vi "Update Gate Parameters Visibility v2.vi"(7 "Edit User-defined Gate":refnum<vi>, 10 "error in (no error)":errorcluster, 11 "Phasor Explorer Gate Parameters in":refnum<vi>) -> (2 "error out":errorcluster, 3 "Phasor Explorer Gate Parameters out":refnum<vi>)   [LabVIEW 2019]
uses:
  Phasor Explorer Gate Parameters.ctl
  Gate Type.ctl
panel:
  in  "Type of User-defined Function":enum32{"Gate", "IRF"}(radio)
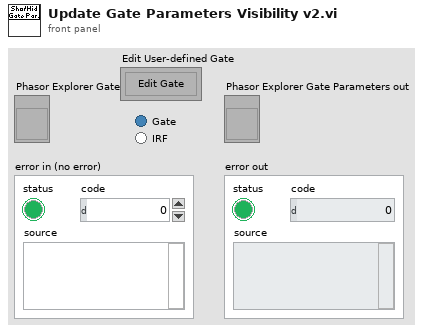
[diagram p1: front panel]
types:
  T1 = typedef "Phasor Explorer Gate Parameters.ctl" = cluster{"First Gate Start":dbl[unit], "Use Gate Center":bool, "Gate Width":dbl[unit], "Gate Step":dbl[unit], "# Gates":dbl, "Gate Type":T2, "Edge Width":dbl[unit], "Top Slope":dbl[unit], "Reversed Sawtooth?":bool, "Analytical Computation":bool, "Integration":enum32{"Item 0", "Item 1"}, "Tolerance":dbl, "# Steps":dbl, "Type of User-defined Function":enum32{"Gate", "IRF"}, "Use Gate Step":bool}
  T2 = typedef "Gate Type.ctl" = enum16{"Square", "Finite Edge Square", "Finite Edge, Tilted Top Square", "Triangle", "Sawtooth", "User-defined"}
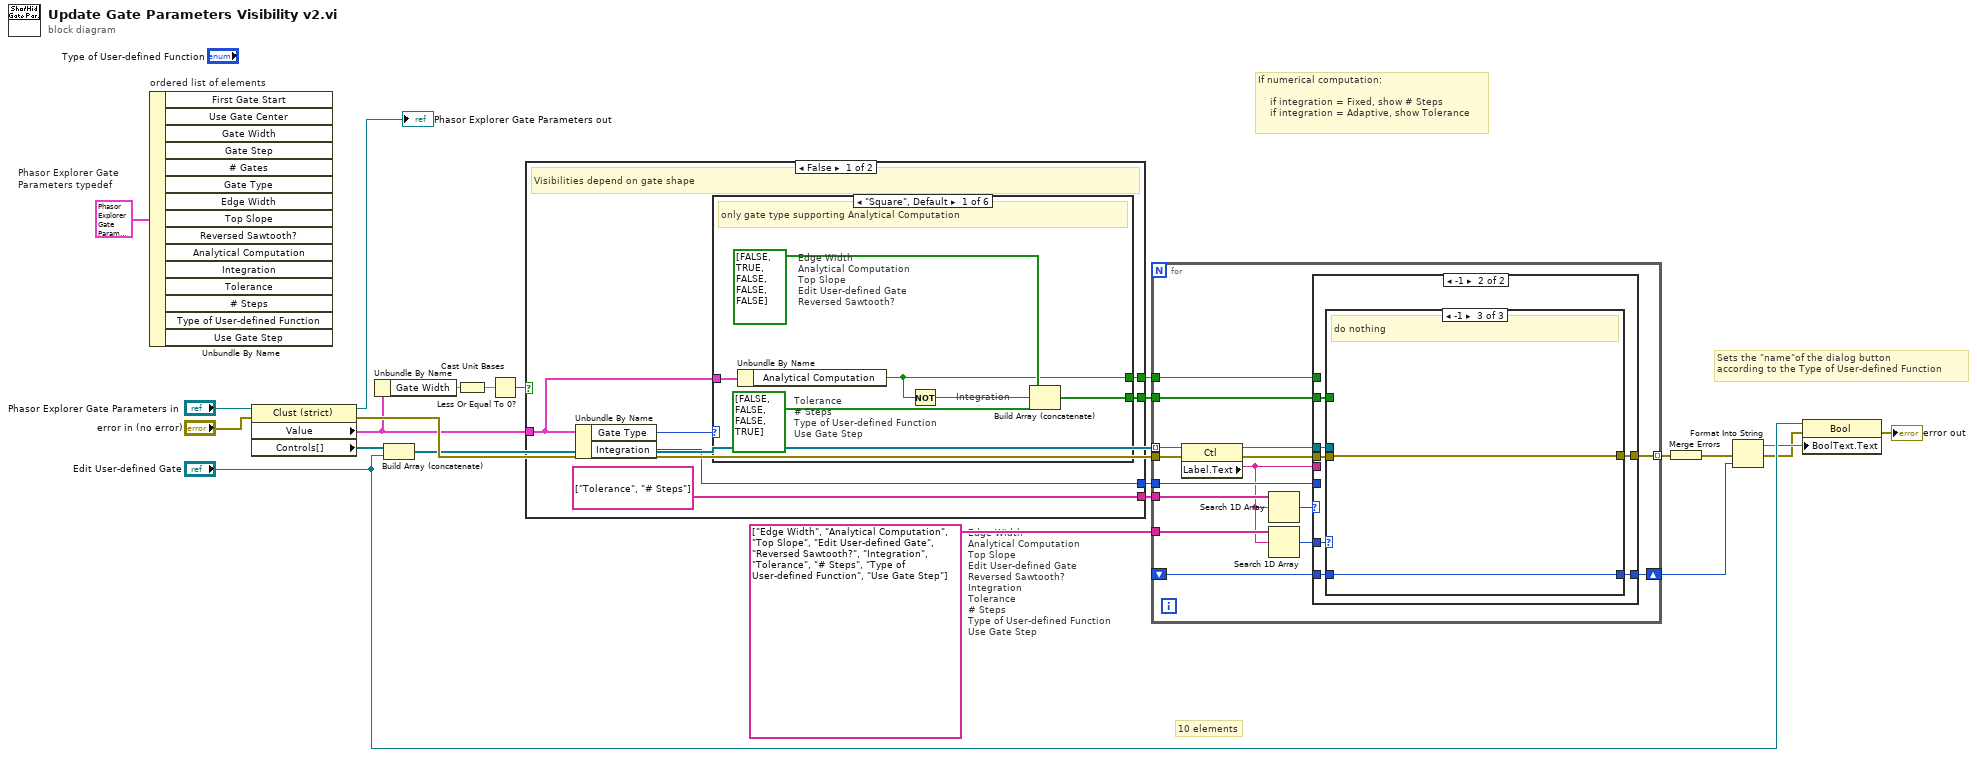
[diagram p0: block diagram]
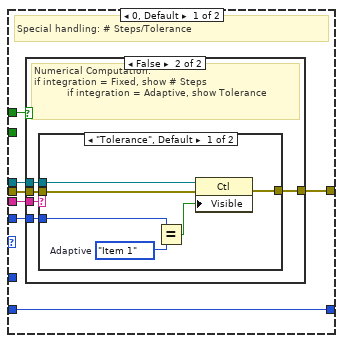
[diagram p2: hidden frame]
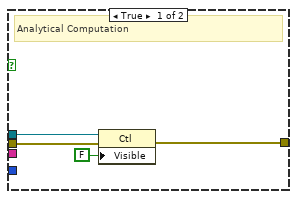
[diagram p3: hidden frame]
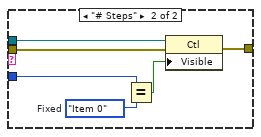
[diagram p4: hidden frame]
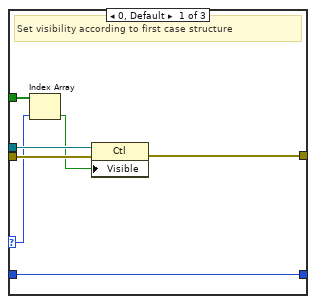
[diagram p5: hidden frame]
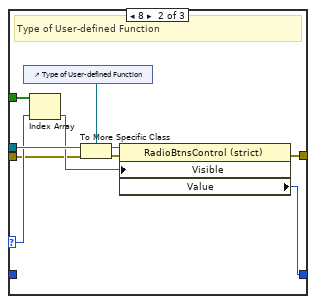
[diagram p6: hidden frame]
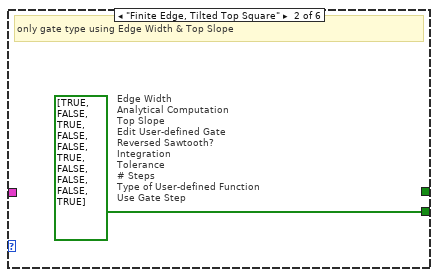
[diagram p7: hidden frame]
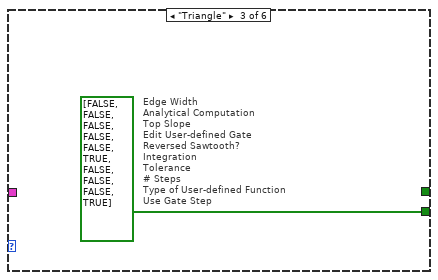
[diagram p8: hidden frame]
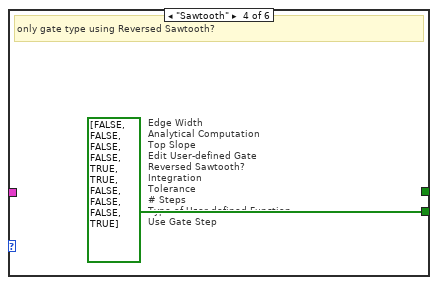
[diagram p9: hidden frame]
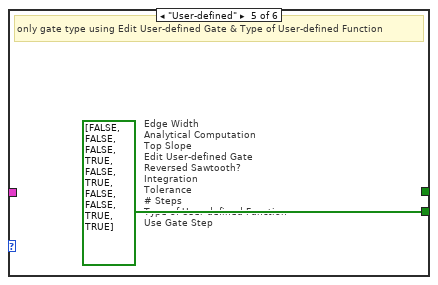
[diagram p10: hidden frame]
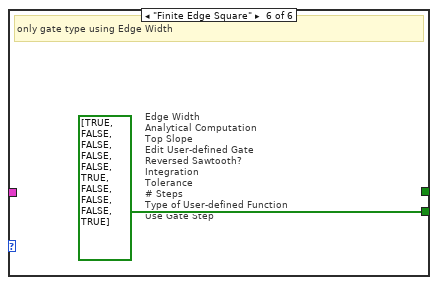
[diagram p11: hidden frame]
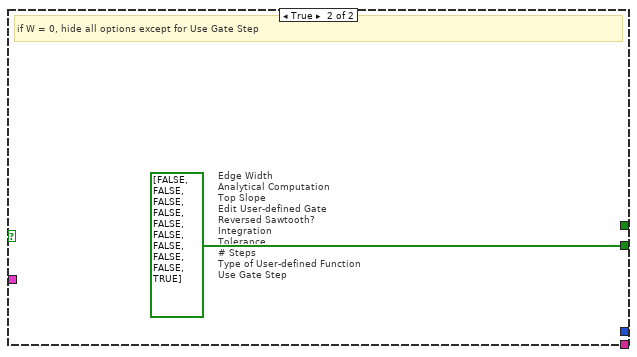
[diagram p12: hidden frame]
diagram:
  w2 = T1 {"First Gate Start"=0.0, "Use Gate Center"=FALSE, "Gate Width"=0.0, "Gate Step"=0.0, "# Gates"=1.0, "Gate Type"=enum."Square", "Edge Width"=0.0, "Top Slope"=0.0, "Reversed Sawtooth?"=FALSE, "Analytical Computation"=FALSE, "Integration"=enum."Item 0", "Tolerance"=1.0, "# Steps"=1.0, "Type of User-defined Function"=enum."Gate", "Use Gate Step"=FALSE}  # Phasor Explorer Gate Parameters typedef
  # "Sets the \"name\"of the dialog button\naccording to the Type of User-defined Function"
  # "If numerical computation:\n\n    if integration = Fixed, show # Steps\n    if integration = Adaptive, show Tolerance"
  # "Edge Width\nAnalytical Computation\nTop Slope\nEdit User-defined Gate\nReversed Sawtooth?\nIntegration\nTolerance\n# Steps\nType of User-defined Function\nUse Gate Step"
  # "10 elements"
  n1 = Unbundle By Name "ordered list of elements"(w2) -> ()  [unwired: 15 out]
  n2 = property class="Clust (strict)"(reference="Phasor Explorer Gate Parameters in", error in="error in (no error)") -> (reference out=→"Phasor Explorer Gate Parameters out":refnum<vi>, error out=w18:errorcluster, "Value"=w15:T1, "Controls[]"=w19:refnum<vi>[])
  n3 = Unbundle By Name(w15) -> ("Gate Width"=w14:dbl[unit])
  n4 = Build Array (concatenate)(w19, "Edit User-defined Gate") -> (w11:refnum<vi>[])
  n5 = Cast Unit Bases(0:w14) -> (2:w13:dbl)  [unwired: 1 in]
  n6 = Less Or Equal To 0?(x=w13) -> (x <= 0?=w12:bool)
  n7 = case shown="False" w12 {
    tunnel: w15 -> [w28 _]
    tunnel: [w27 bool[] [FALSE, FALSE, FALSE, FALSE, FALSE, FALSE, FALSE, FALSE, FALSE, TRUE] ("Label.Text")] -> w17
    tunnel: [w26 _] -> w10
    tunnel: [w25 _] -> w3
    tunnel: [string[] ["Tolerance", "# Steps"] ("Label.Text") _] -> w1
    frame False {
      # "Visibilities depend on gate shape"
      n8 = Unbundle By Name(w28) -> ("Gate Type"=w29:T2, "Integration"=w25:enum32{"Item 0", "Item 1"})
      n9 = case shown="\"Square\", Default" w29 {
        tunnel: w28 -> [w35 _ _ _ _ _]
        tunnel: [w33 bool[] [TRUE, FALSE, TRUE, FALSE, FALSE, TRUE, FALSE, FALSE, FALSE, TRUE] ("Label.Text") bool[] [FALSE, FALSE, FALSE, FALSE, FALSE, TRUE, FALSE, FALSE, FALSE, TRUE] ("Label.Text") bool[] [FALSE, FALSE, FALSE, FALSE, TRUE, TRUE, FALSE, FALSE, FALSE, TRUE] ("Label.Text") bool[] [FALSE, FALSE, FALSE, TRUE, FALSE, TRUE, FALSE, FALSE, TRUE, TRUE] ("Label.Text") bool[] [TRUE, FALSE, FALSE, FALSE, FALSE, TRUE, FALSE, FALSE, FALSE, TRUE] ("Label.Text")] -> w27
        tunnel: [w31 _ _ _ _ _] -> w26
        frame "Square", Default {
          # "Integration"
          # "Tolerance\n# Steps\nType of User-defined Function\nUse Gate Step"
          # "Edge Width\nAnalytical Computation\nTop Slope\nEdit User-defined Gate\nReversed Sawtooth?"
          # "only gate type supporting Analytical Computation"
          n10 = Unbundle By Name(w35) -> ("Analytical Computation"=w31:bool)
          n11 = Not(x=w31) -> (.not. x?=w32:bool)
          n12 = Build Array (concatenate)(bool[] [FALSE, TRUE, FALSE, FALSE, FALSE] ("Label.Text"), w32, bool[] [FALSE, FALSE, FALSE, TRUE] ("Label.Text")) -> (w33:bool[])
        }
        frame "Finite Edge, Tilted Top Square" {
          # "Edge Width\nAnalytical Computation\nTop Slope\nEdit User-defined Gate\nReversed Sawtooth?\nIntegration\nTolerance\n# Steps\nType of User-defined Function\nUse Gate Step"
          # "only gate type using Edge Width & Top Slope"
        }
        frame "Triangle" {
          # "Edge Width\nAnalytical Computation\nTop Slope\nEdit User-defined Gate\nReversed Sawtooth?\nIntegration\nTolerance\n# Steps\nType of User-defined Function\nUse Gate Step"
        }
        frame "Sawtooth" {
          # "Edge Width\nAnalytical Computation\nTop Slope\nEdit User-defined Gate\nReversed Sawtooth?\nIntegration\nTolerance\n# Steps\nType of User-defined Function\nUse Gate Step"
          # "only gate type using Reversed Sawtooth?"
        }
        frame "User-defined" {
          # "Edge Width\nAnalytical Computation\nTop Slope\nEdit User-defined Gate\nReversed Sawtooth?\nIntegration\nTolerance\n# Steps\nType of User-defined Function\nUse Gate Step"
          # "only gate type using Edit User-defined Gate & Type of User-defined Function"
        }
        frame "Finite Edge Square" {
          # "Edge Width\nAnalytical Computation\nTop Slope\nEdit User-defined Gate\nReversed Sawtooth?\nIntegration\nTolerance\n# Steps\nType of User-defined Function\nUse Gate Step"
          # "only gate type using Edge Width"
        }
      }
    }
    frame True {
      # "Edge Width\nAnalytical Computation\nTop Slope\nEdit User-defined Gate\nReversed Sawtooth?\nIntegration\nTolerance\n# Steps\nType of User-defined Function\nUse Gate Step"
      # "if W = 0, hide all options except for Use Gate Step"
    }
  }
  n13 = for {
    tunnel: string[] ["Edge Width", "Analytical Computation", "Top Slope", "Edit User-defined Gate", "Reversed Sawtooth?", "Integration", "Tolerance", "# Steps", "Type of User-defined Function", "Use Gate Step"] ("Label.Text") -> [w56]
    tunnel: w11 -> [w55] mode=indexing
    tunnel: w18 -> [w54]
    tunnel: w17 -> [w53]
    tunnel: [w51] -> w16 mode=indexing
    tunnel: w10 -> [w48]
    shift-right: [w47] -> w7
    shift-left: _ -> [w46]
    tunnel: w3 -> [w45]
    tunnel: w1 -> [w44]
    n14 = property class="Ctl"(reference=w55, error in=w54) -> (reference out=w50:refnum<vi>, error out=w49:errorcluster, "Label.Text"=w42:string)
    n15 = Search 1D Array(1D array=w44, element=w42) -> (index of element=w43:i32)  [unwired: 1 in]
    n16 = Search 1D Array(1D array=w56, element=w42) -> (index of element=w52:i32)  [unwired: 1 in]
    n17 = case shown="-1" w43 {
      tunnel: w53 -> [_ w91]
      tunnel: w52 -> [_ w90]
      tunnel: [w63 w89] -> w51
      tunnel: w50 -> [w62 w88]
      tunnel: w49 -> [w61 w87]
      tunnel: w48 -> [w59 _]
      tunnel: [w60 w86] -> w47
      tunnel: w46 -> [w60 w85]
      tunnel: w45 -> [w57 _]
      tunnel: w42 -> [w58 _]
      frame 0, Default {
        # "Special handling: # Steps/Tolerance"
        n18 = case shown="False" w59 {
          tunnel: [w67 w72] -> w63
          tunnel: w62 -> [w66 w71]
          tunnel: w61 -> [w65 w70]
          tunnel: w58 -> [_ w69]
          tunnel: w57 -> [_ w68]
          frame True {
            # "Analytical Computation"
            n19 = property class="Ctl"(reference=w66, error in=w65, "Visible"=FALSE) -> (error out=w67:errorcluster)  [unwired: 1 out]
          }
          frame False {
            # "Numerical Computation:\nif integration = Fixed, show # Steps\n           if integration = Adaptive, show Tolerance"
            n20 = case shown="\"Tolerance\", Default" w69 {
              tunnel: [w78 w84] -> w72
              tunnel: w71 -> [w77 w83]
              tunnel: w70 -> [w76 w82]
              tunnel: w68 -> [w75 w81]
              frame "Tolerance", Default {
                w74 = enum32{"Item 0", "Item 1"}."Item 1"  # Adaptive
                n21 = Equal?(x=w75, y=w74) -> (x = y?=w73:bool)
                n22 = property class="Ctl"(reference=w77, error in=w76, "Visible"=w73) -> (error out=w78:errorcluster)  [unwired: 1 out]
              }
              frame "# Steps" {
                w80 = enum32{"Item 0", "Item 1"}."Item 0"  # Fixed
                n23 = Equal?(x=w81, y=w80) -> (x = y?=w79:bool)
                n24 = property class="Ctl"(reference=w83, error in=w82, "Visible"=w79) -> (error out=w84:errorcluster)  [unwired: 1 out]
              }
            }
          }
        }
      }
      frame -1 {
        n25 = case shown="-1" w90 {
          selector: w90 -> [w95 w106 _]
          tunnel: w88 -> [w98 w108 _]
          tunnel: w87 -> [w97 w102 w110]
          tunnel: w91 -> [w96 w107 _]
          tunnel: [w93 w104 w110] -> w89
          tunnel: [w92 w99 w109] -> w86
          tunnel: w85 -> [w92 _ w109]
          frame 0, Default {
            # "Set visibility according to first case structure"
            n26 = Index Array(array=w96, index=w95) -> (element=w94:bool)
            n27 = property class="Ctl"(reference=w98, error in=w97, "Visible"=w94) -> (error out=w93:errorcluster)  [unwired: 1 out]
          }
          frame 8 {
            # "Type of User-defined Function"
            n28 = control-ref of="Type of User-defined Function"() -> (w100:refnum<vi>)
            n29 = Index Array(array=w107, index=w106) -> (element=w105:bool)
            n30 = To More Specific Class(target class=w100, reference=w108, error in=w102) -> (specific class reference=w103:refnum<vi>, error out=w101:errorcluster)
            n31 = property class="RadioBtnsControl (strict)"(reference=w103, error in=w101, "Visible"=w105) -> (error out=w104:errorcluster, "Value"=w99:enum32{"Gate", "IRF"})  [unwired: 1 out]
          }
          frame -1 {
            # "do nothing"
          }
        }
      }
    }
  }
  n32 = Merge Errors(w16) -> (w5:errorcluster)
  n33 = Format Into String(error in=w5, w7) -> (resulting string=w6:string, error out=w4:errorcluster)  [unwired: 2 in]
  n34 = property class="Bool"(reference="Edit User-defined Gate", error in=w4, "BoolText.Text"=w6) -> (error out=→"error out":errorcluster)  [unwired: 1 out]
